vi "Compile Channel States.vi"(8 "error in (no error)":errorcluster, 9 "Channel States":T4, 10 "Communication Configuration":T1, 11 "Compiled Connections Buffer in":T2[](array[typedef])) -> (0 "error out":errorcluster, 2 "Value-Connections Map":T3, 3 "Compiled Connections Buffer out":T2[](array[typedef]))   [LabVIEW 2020, in "Routing and Faulting System Explorer.lvlib"]
uses:
  Routing and Faulting System Explorer.lvlib
  Shared/Channel States.ctl
  Shared/Routing State.ctl
  Shared/Connection.ctl
  Shared/Value-Connections Map.ctl
  Shared/Compiled Connection.ctl
  Shared/Communication Configuration.ctl
  Shared/Routing and Faulting Shared.lvlib
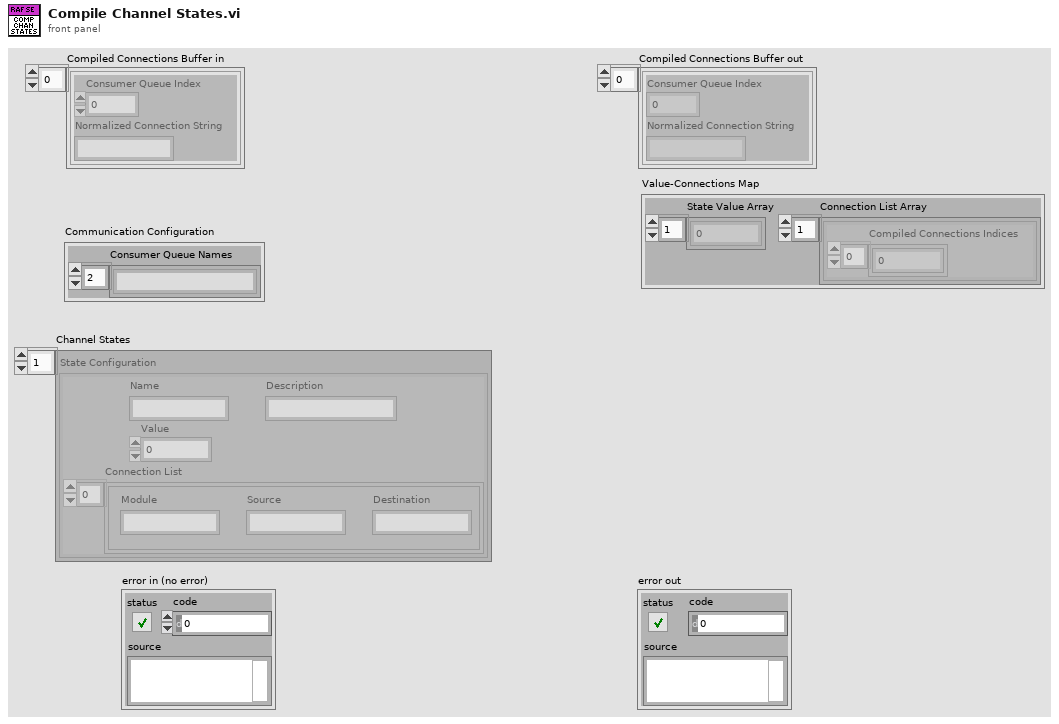
[diagram p1: front panel]
types:
  T1 = typedef "Routing and Faulting Shared.lvlib/Communication Configuration.ctl" = cluster{"Consumer Queue Names":string[]}
  T2 = typedef "Routing and Faulting Shared.lvlib/Compiled Connection.ctl" = cluster{"Consumer Queue Index":i32, "Normalized Connection String":string}
  T3 = typedef "Routing and Faulting Shared.lvlib/Value-Connections Map.ctl" = cluster{"State Value Array":i32[], "Connection List Array":cluster{"Compiled Connections Indices":i32[]}[]}
  T4 = typedef "Routing and Faulting Shared.lvlib/Channel States.ctl" = T5[]
  T5 = typedef "Routing and Faulting Shared.lvlib/Routing State.ctl" = cluster{"Name":string, "Description":string, "Value":i32, "Connection List":T6[]}
  T6 = typedef "Routing and Faulting Shared.lvlib/Connection.ctl" = cluster{"Module":string, "Source":string, "Destination":string}
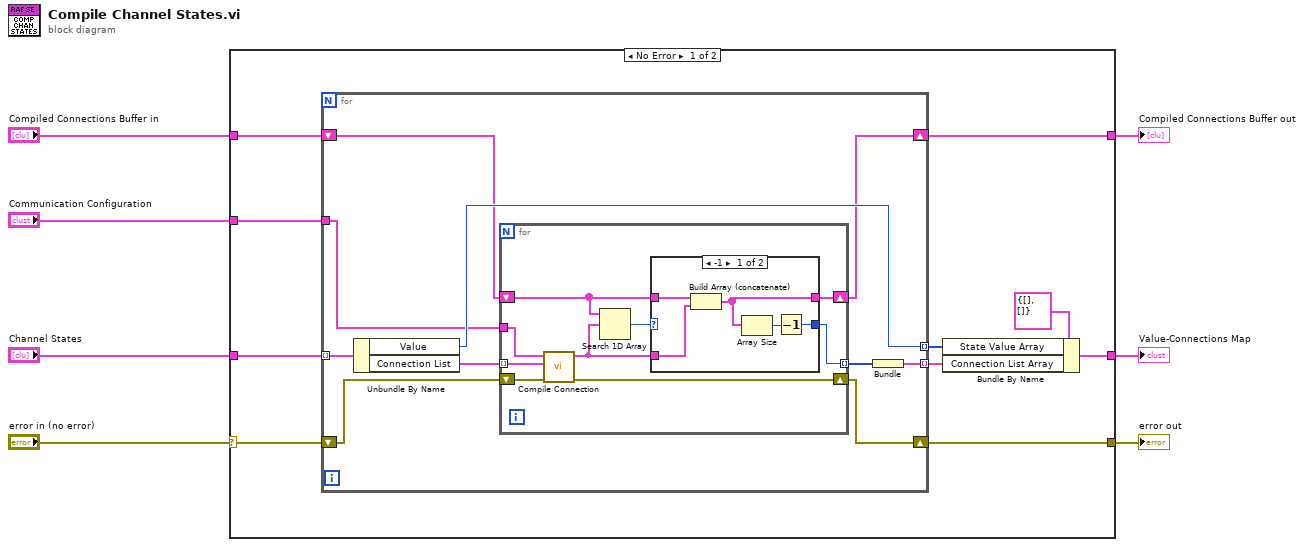
[diagram p0: block diagram]
diagram:
  n1 = case shown="No Error" "error in (no error)" {
    selector: "error in (no error)" -> [w15 w45]
    tunnel: "Channel States" -> [w17 _]
    tunnel: [w16 _] -> w4
    tunnel: [w14 w45] -> w5
    tunnel: "Compiled Connections Buffer in" -> [w11 w44]
    tunnel: "Communication Configuration" -> [w10 _]
    tunnel: [w9 w44] -> w1
    frame No Error {
      n2 = for {
        tunnel: w17 -> [w27] mode=indexing
        tunnel: [w26] -> w12 mode=indexing
        shift-right: [w18] -> w14
        shift-left: w15 -> [w19]
        tunnel: w10 -> [w23]
        shift-right: [w22] -> w9
        shift-left: w11 -> [w24]
        tunnel: [w20] -> w8 mode=indexing
        n3 = Unbundle By Name(w27) -> ("Value"=w26:i32, "Connection List"=w25:T6[])
        n4 = for {
          tunnel: w25 -> [w36] mode=indexing
          tunnel: w23 -> [w35]
          shift-right: [w31] -> w22
          shift-left: w24 -> [w33]
          tunnel: [w30] -> w21 mode=indexing
          shift-right: [w28] -> w18
          shift-left: w19 -> [w29]
          n5 = call "Compile Connection.vi"("error in (no error)"=w29, "Connection"=w36, "Communication Configuration"=w35) -> ("error out"=w28:errorcluster, "Compiled Connection"=w32:T2)  [unwired: 7 in]
          n6 = Search 1D Array(1D array=w33, element=w32) -> (index of element=w34:i32)  [unwired: 1 in]
          n7 = case shown="-1" w34 {
            selector: w34 -> [_ w42]
            tunnel: w33 -> [w39 w43]
            tunnel: w32 -> [w41 _]
            tunnel: [w38 w43] -> w31
            tunnel: [w37 w42] -> w30
            frame -1 {
              n8 = Build Array (concatenate)(w39, w41) -> (w38:T2[])
              n9 = Array Size(array=w38) -> (size(s)=w40:i32)
              n10 = Decrement(x=w40) -> (x-1=w37:i32)
            }
            frame Default {
            }
          }
        }
        n11 = Bundle(w21) -> (w20:cluster{i32[]})  [unwired: 1 in]
      }
      n12 = Bundle By Name(cluster=T3 {"State Value Array"=[], "Connection List Array"=[]} ("Value-Connections Map"), "State Value Array"=w12, "Connection List Array"=w8) -> (w16:T3)
    }
    frame Error {
    }
  }
  "error out" <- w5
  "Value-Connections Map" <- w4
  "Compiled Connections Buffer out" <- w1
